vi "DBL Array to Hex.vi"(11 "Array":dbl[](array[numeric])) -> ()   [LabVIEW 2020]
panel:
  out "String":string
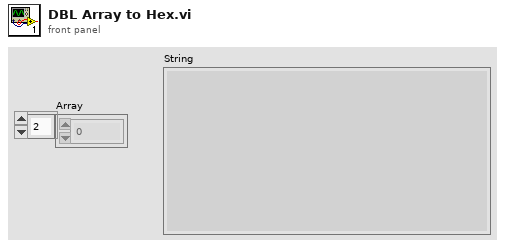
[diagram p1: front panel]
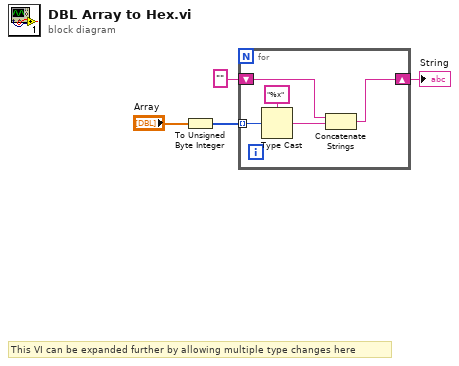
[diagram p0: block diagram]
diagram:
  # "This VI can be expanded further by allowing multiple type changes here"
  n1 = To Unsigned Byte Integer(number="Array") -> (unsigned 8bit integer=w1:u8[])
  n2 = for {
    shift-right: [w5] -> w2
    shift-left: "" -> [w6]
    tunnel: w1 -> [w8] mode=indexing
    n3 = Type Cast(type="%x", x=w8) -> (*(type *) &x=w7:string)
    n4 = Concatenate Strings(w6, w7) -> (w5:string)
  }
  "String" <- w2
